vi "Read N Packets.vi"(7 "Timestamps and Lengths Alloc":T1, 8 "error in (no error)":errorcluster, 9 "Num Packets to Read":i32=128, 10 "capture_data_buffer":string, 11 "pcap reference":u64) -> (0 "error out":errorcluster, 1 "Num Packets Read":i32, 2 "capture_data out":string, 3 "pcap reference out":u64, 4 "timeout":bool, 5 "Timestamps and Lengths out":T1, 6 "EOF":bool)   [LabVIEW 2025, in "Automotive Ethernet Bus Monitor UI.lvlib" / "lvwpcap.lvlib"]
doc: "This VI reads an ethernet packet. It outputs the packet in the form of a raw string."
uses:
  lvwpcap.lvlib
  lvwpcap.dll
  types/Capture Legnths.ctl
  types/Timestamps and Lengths.ctl
panel:
  # "Select Help»Show Context Help and move the cursor over the VI icon to display help for this VI."
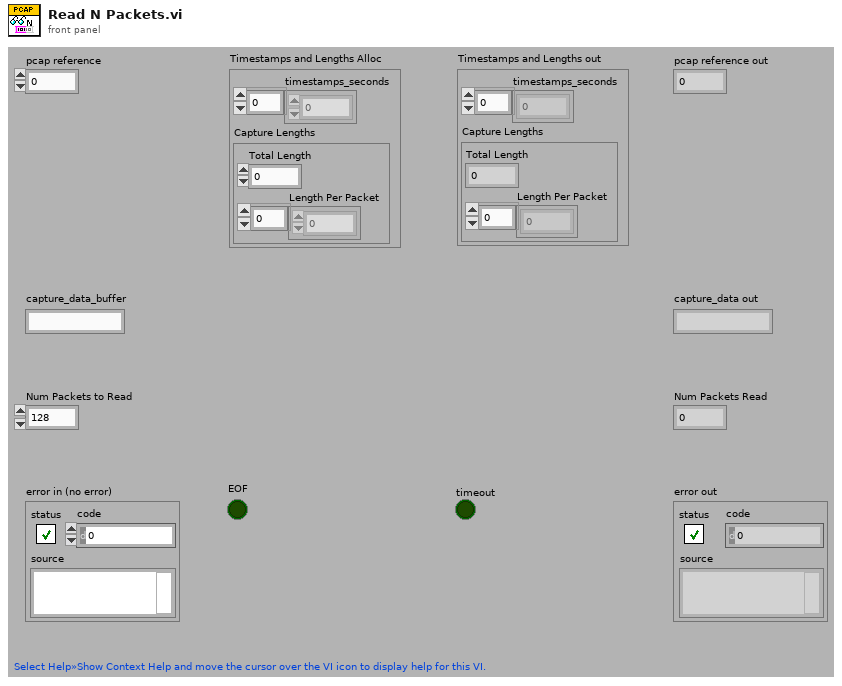
[diagram p1: front panel]
types:
  T1 = typedef "Automotive Ethernet Bus Monitor UI.lvlib/lvwpcap.lvlib/Timestamps and Lengths.ctl" = cluster{"timestamps_seconds":dbl[], "Capture Lengths":T2}
  T2 = typedef "Automotive Ethernet Bus Monitor UI.lvlib/lvwpcap.lvlib/Capture Legnths.ctl" = cluster{"Total Length":u32, "Length Per Packet":u32[]}
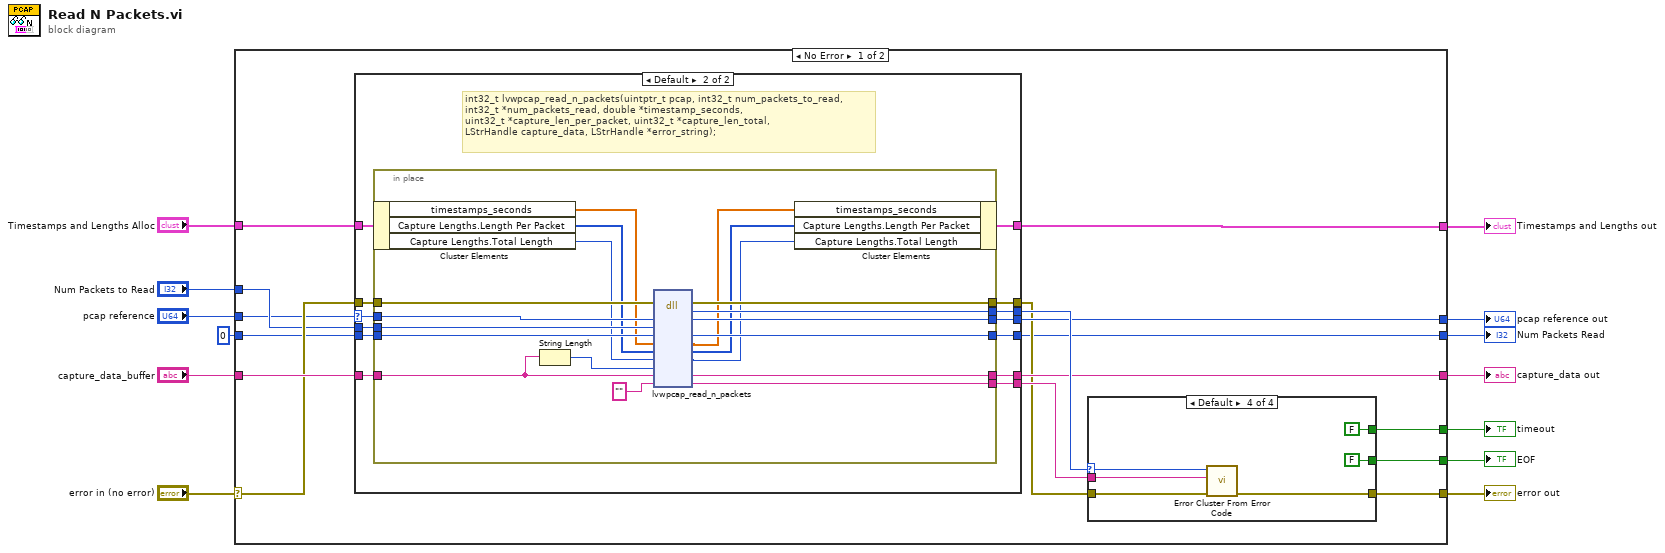
[diagram p0: block diagram]
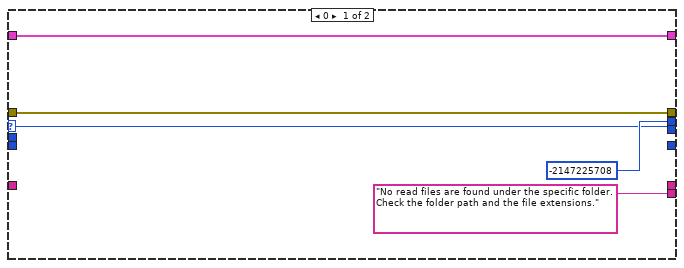
[diagram p2: hidden frame]
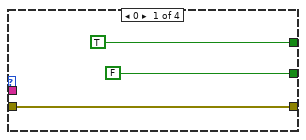
[diagram p3: hidden frame]
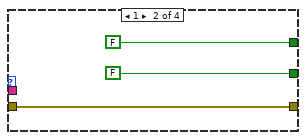
[diagram p4: hidden frame]
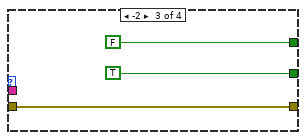
[diagram p5: hidden frame]
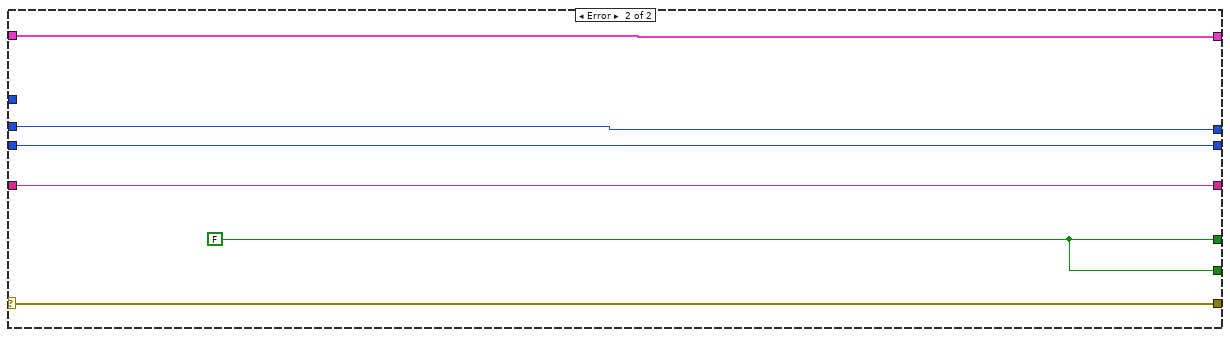
[diagram p6: hidden frame]
diagram:
  n1 = case shown="No Error" "error in (no error)" {
    selector: "error in (no error)" -> [w21 w87]
    tunnel: [w29 w87] -> w13
    tunnel: [w26 w84] -> w11
    tunnel: "pcap reference" -> [w14 w86]
    tunnel: "capture_data_buffer" -> [w25 w85]
    tunnel: [w24 w86] -> w8
    tunnel: [w23 w85] -> w7
    tunnel: [w20 w84] -> w6
    tunnel: "Num Packets to Read" -> [w19 _]
    tunnel: [w18 w83] -> w4
    tunnel: 0 ("num_packets_read") -> [w17 w83]
    tunnel: "Timestamps and Lengths Alloc" -> [w16 w82]
    tunnel: [w15 w82] -> w1
    frame No Error {
      n2 = case shown="Default" w14 {
        selector: w14 -> [w30 w35]
        tunnel: [-2147225708 ("return type") w47] -> w28
        tunnel: ["No read files are found under the specific folder. Check the folder path and the file extensions." ("error_string") w46] -> w27
        tunnel: w25 -> [_ w45]
        tunnel: [w30 w44] -> w24
        tunnel: [_ w43] -> w23
        tunnel: [w34 w42] -> w22
        tunnel: w21 -> [w34 w41]
        tunnel: w19 -> [_ w40]
        tunnel: [_ w39] -> w18
        tunnel: w17 -> [_ w38]
        tunnel: w16 -> [w33 w37]
        tunnel: [w33 w36] -> w15
        frame 0 {
        }
        frame Default {
          # "int32_t lvwpcap_read_n_packets(uintptr_t pcap, int32_t num_packets_to_read, \nint32_t *num_packets_read, double *timestamp_seconds, \nuint32_t *capture_len_per_packet, uint32_t *capture_len_total, \nLStrHandle capture_data, LStrHandle *error_string);"
          n3 = in-place {
            in-place-border: [w66] -> w47
            in-place-border: [w65] -> w46
            in-place-border: w35 -> [w64]
            in-place-border: w45 -> [w49]
            in-place-border: [w63] -> w44
            in-place-border: [w62] -> w43
            in-place-border: [w61] -> w42
            in-place-border: w41 -> [w60]
            in-place-border: w40 -> [w59]
            in-place-border: [w58] -> w39
            in-place-border: w38 -> [w57]
            n4 = in-place-cluster #1(w37) -> ("timestamps_seconds"=w56:dbl[], "Capture Lengths.Length Per Packet"=w54:u32[], "Capture Lengths.Total Length"=w52:u32)
            n5 = String Length(string=w49) -> (length=w48:i32)
            n6 = dll-call lib="lvwpcap.*" fn="lvwpcap_read_n_packets"(error in=w60, "pcap"=w64, "num_packets_to_read"=w59, "num_packets_read"=w57, "timestamp_seconds"=w56, "capture_len_per_packet"=w54, "capture_len_total"=w52, "capture_data_size"=w48, "capture_data"=w49, "error_string"="") -> (error out=w61:errorcluster, "return type"=w66:i32, "pcap"=w63:u64, "num_packets_read"=w58:i32, "timestamp_seconds"=w55:dbl[], "capture_len_per_packet"=w53:u32[], "capture_len_total"=w51:u32, "capture_data"=w62:string, "error_string"=w65:string)  [unwired: 4 in, 1 out]
            n7 = in-place-cluster #1("timestamps_seconds"=w55, "Capture Lengths.Length Per Packet"=w53, "Capture Lengths.Total Length"=w51) -> (w36:T1)
          }
        }
      }
      n8 = case shown="Default" w28 {
        selector: w28 -> [_ _ _ w77]
        tunnel: w27 -> [_ _ _ w76]
        tunnel: w22 -> [w69 w72 w74 w79]
        tunnel: [w69 w72 w74 w78] -> w29
        tunnel: [TRUE FALSE FALSE FALSE] -> w26
        tunnel: [FALSE FALSE TRUE FALSE] -> w20
        frame 0 {
        }
        frame 1 {
        }
        frame -2 {
        }
        frame Default {
          n9 = call <vilib>:"Error Cluster From Error Code.vi"("error in (no error)"=w79, "error message (\"\")"=w76, "error code (0)"=w77) -> ("error out"=w78:errorcluster)  [unwired: 6 in]
        }
      }
    }
    frame Error {
      w84 = FALSE
    }
  }
  "error out" <- w13
  "timeout" <- w11
  "pcap reference out" <- w8
  "capture_data out" <- w7
  "EOF" <- w6
  "Num Packets Read" <- w4
  "Timestamps and Lengths out" <- w1
